vi "Configure Multi Eval Meas All Results Enabled.vi"(7 "Enable All Results":bool[](array[boolean]), 8 "error in (no error)":errorcluster, 10 "Instance (1)":i32=1, 11 "VISA resource name":refnum<visa-resource-name>) -> (0 "error out":errorcluster, 3 "VISA resource name out":refnum<visa-resource-name>)   [LabVIEW 2020, in "Rohde&Schwarz CMP LR WPAN Measurement.lvlib"]
doc: "Enables or disables the evaluation of results in the multi-evaluation measurement. Combines all other CONFigure:WPAN:MEAS<i>:MEValuation:RESult... commands.\n\nOrder of elements in an array:\n<PvT>, <PowerScalars>, <EVMChip>, <ModScalars>, <PowSpecDensity>[, <IQConstellation>]\n\nParameters:\n<PvT> - Enables or disables Power vs time results\n\n<PowerScalars> - Enables or disables Statistical power results\n\n<EVMChip> - Enables or disables Error vector magnitude vs chip\n\n<ModScalars> - Enables or disables Statistical modulation results\n\n<PowSpecDensity> - Enables or disables Power spectral density results\n\n<IQConstellation> - Enables or disables IQ constellation results\n\nAttribute:\n-\n\nRemote-control command:\nCONFigure:WPAN:MEAS<i>:MEValuation:RESult[:ALL]"
uses:
  <instrlib>/Rohde&Schwarz CMP LR WPAN Measurement/Rohde&Schwarz CMP LR WPAN Measurement.lvlib
  <instrlib>/Rohde&Schwarz CMP LR WPAN Measurement/Private/rsidr_core.llb/rsidr_core.lvlib
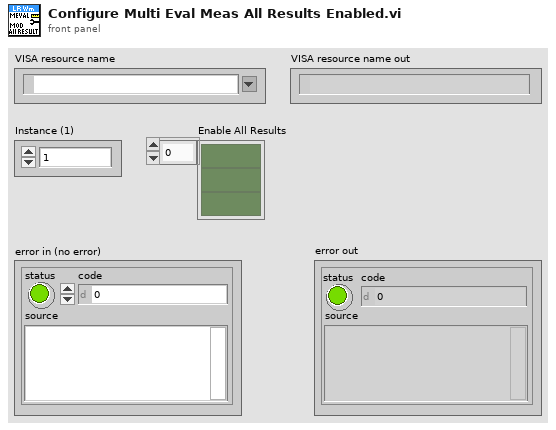
[diagram p1: front panel]
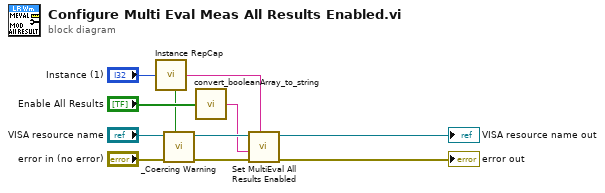
[diagram p0: block diagram]
diagram:
  n1 = call <instrlib>:"Instance RepCap.vi"("Instance In"="Instance (1)") -> ("In Range?"=w8:bool, "RepCap Identifier Out"=w7:string)  [unwired: 1 in]
  n2 = call <instrlib>:"_Coercing Warning.vi"("In Range?"=w8, "error in (no error)"="error in (no error)", "VISA resource name"="VISA resource name") -> ("error out"=w4:errorcluster, "VISA resource name out"=w3:refnum<visa-resource-name>)  [unwired: 7 in]
  n3 = call <instrlib>:"convert_booleanArray_to_string.vi"("Boolean array in"="Enable All Results") -> ("string out"=w1:string)  [unwired: 4 in]
  n4 = call "Set MultiEval All Results Enabled"("Repeated Capabilities"=w7, "error in (no error)"=w4, "MultiEval All Results Enabled ()"=w1, "instrument handle"=w3) -> ("error out"=→"error out":errorcluster, "instrument handle out"=→"VISA resource name out":refnum<visa-resource-name>)  [unwired: 6 in]
